vi "Determine Warnings (Challenge).vi"() -> ()   [LabVIEW 2014]
panel:
  out "Warning?":bool
  out "Warning Text":string
  in  "Min Temp":dbl
  in  "Max Temp":dbl
  in  "Current Temp":dbl
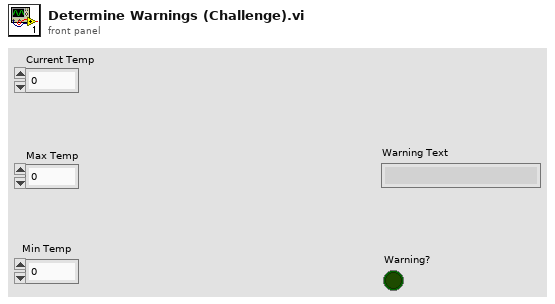
[diagram p1: front panel]
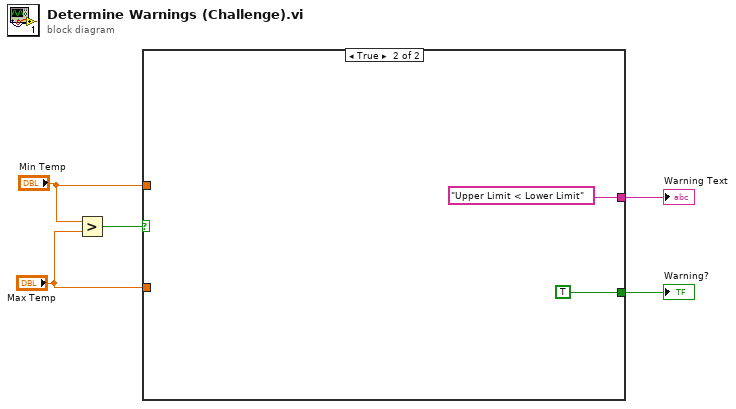
[diagram p0: block diagram]
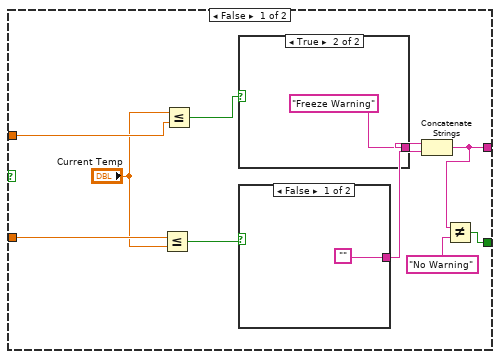
[diagram p2: hidden frame]
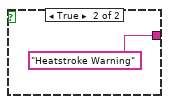
[diagram p3: hidden frame]
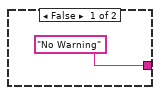
[diagram p4: hidden frame]
diagram:
  n1 = Greater?(x="Min Temp", y="Max Temp") -> (0:w5:bool)
  n2 = case shown="True" w5 {
    tunnel: [w7 "Upper Limit < Lower Limit"] -> w1
    tunnel: [w8 TRUE] -> w4
    tunnel: "Max Temp" -> [w15 _]
    tunnel: "Min Temp" -> [w14 _]
    frame False {
      n3 = Less Or Equal?(x=w15, y="Current Temp") -> (x <= y?=w11:bool)
      n4 = Less Or Equal?(x="Current Temp", y=w14) -> (x <= y?=w12:bool)
      n5 = case shown="True" w12 {
        tunnel: ["No Warning" "Freeze Warning"] -> w10
        frame False {
        }
        frame True {
        }
      }
      n6 = case shown="False" w11 {
        tunnel: ["" "Heatstroke Warning"] -> w9
        frame False {
        }
        frame True {
        }
      }
      n7 = Concatenate Strings(w10, w9) -> (w7:string)
      n8 = Not Equal?(x=w7, y="No Warning") -> (x != y?=w8:bool)
    }
    frame True {
    }
  }
  "Warning Text" <- w1
  "Warning?" <- w4
